vi "detection_gate.vi"(8 "Error_in":errorcluster, 9 "read_width_us":dbl, 10 "pulse_period_us":dbl[](array[numeric]), 11 "correction_us":dbl) -> (0 "start_read":u32[](array[numeric]), 1 "stop_read":u32[](array[numeric]))   [LabVIEW 2018]
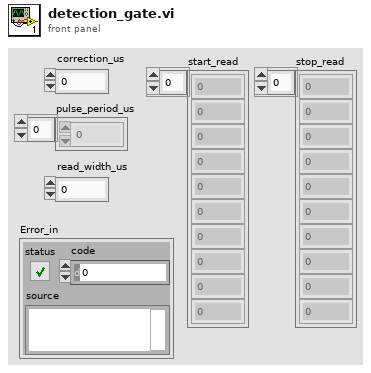
[diagram p1: front panel]
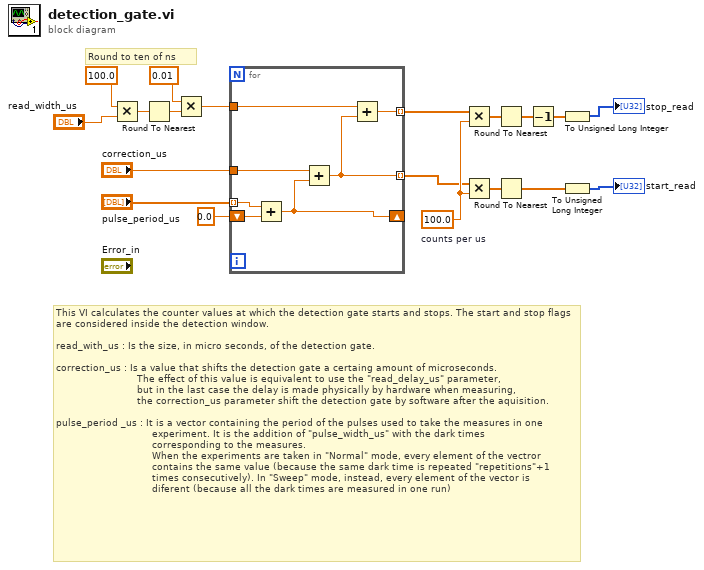
[diagram p0: block diagram]
diagram:
  w19 = 100.0  # counts per us
  # "This VI calculates the counter values at which the detection gate starts and stops. The start and stop flags are considered inside the detection window.\n\nread_with_us : Is the size, in micro seconds, of the detection gate.\n\ncorrection_us : Is a value that shifts the detection gate a certaing amount of microseconds.\n                           The effect of this value is equivalent to use the \"read_delay_us\" parameter, \n                           but in the last case the delay is made physically by hardware when measuring,\n                           the correction_us parameter shift the detection gate by software after the aquisition.\n\npulse_period _us : It is a vector containing the period of the pulses used to take the measures in one\n                                experiment. It is the addition of \"pulse_width_us\" with the dark times\n                                corresponding to the measures.\n                                When the experiments are taken in \"Normal\" mode, every element of the vectror\n                                contains the same value (because the same dark time is repeated \"repetitions\"+1\n                                times consecutively). In \"Sweep\" mode, instead, every element of the vector is \n                                diferent (because all the dark times are measured in one run)"
  # "Round to ten of ns"
  n1 = Multiply(x=100.0, y="read_width_us") -> (x*y=w7:dbl)
  n2 = Round To Nearest(number=w7) -> (nearest integer value=w6:dbl)
  n3 = Multiply(x=0.01, y=w6) -> (x*y=w2:dbl)
  n4 = for {
    tunnel: [w21] -> w13 mode=indexing
    tunnel: [w22] -> w12 mode=indexing
    tunnel: "pulse_period_us" -> [w26] mode=indexing
    shift-right: [w24] -> _
    shift-left: 0.0 -> [w25]
    tunnel: "correction_us" -> [w23]
    tunnel: w2 -> [w20]
    n5 = Add(x=w26, y=w25) -> (x+y=w24:dbl)
    n6 = Add(x=w23, y=w24) -> (x+y=w22:dbl)
    n7 = Add(x=w20, y=w22) -> (x+y=w21:dbl)
  }
  n8 = Multiply(x=w13, y=w19) -> (x*y=w18:dbl[])
  n9 = Multiply(x=w12, y=w19) -> (x*y=w17:dbl[])
  n10 = Round To Nearest(number=w18) -> (nearest integer value=w15:dbl[])
  n11 = Round To Nearest(number=w17) -> (nearest integer value=w16:dbl[])
  n12 = Decrement(x=w15) -> (x-1=w14:dbl[])
  n13 = To Unsigned Long Integer(number=w14) -> (unsigned 32bit integer=→"stop_read":u32[])
  n14 = To Unsigned Long Integer(number=w16) -> (unsigned 32bit integer=→"start_read":u32[])
